vi "Triggers-Reset soft trigger.vi"(6 "Reset soft. trigger":bool, 8 "error in (no error)":errorcluster, 11 "FPGA Ref":T1) -> (0 "error out":errorcluster)   [LabVIEW 2013]
uses:
  RIG-SPECIFIC FILES/FPGA Refs/FPGA Ref.ctl
  <vilib>/rvi/interface/common/niFpgaWaitOnOcc.vi
  <vilib>/Utility/error.llb/Error Cluster From Error Code.vi
  <vilib>/rvi/errors/niLvFpgaAdjustHostInterfaceError.vi
  <vilib>/rvi/interface/nirviReadWriteControl/nirviReadWriteControl.xnode
  NiFpgaLv.dll
  <vilib>/rvi/interface/Simulation/niFpgaSimulationCallBeginRW.vi
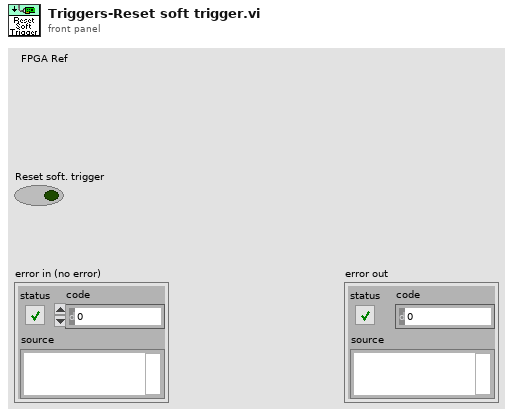
[diagram p1: front panel]
types:
  T1 = typedef "FPGA Ref.ctl" = refnum<k20>
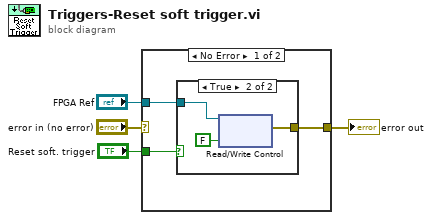
[diagram p0: block diagram]
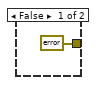
[diagram p2: hidden frame]
diagram:
  n1 = case shown="No Error" "error in (no error)" {
    selector: "error in (no error)" -> [_ w12]
    tunnel: [w5 w12] -> w4
    tunnel: "FPGA Ref" -> [w7 _]
    tunnel: "Reset soft. trigger" -> [w6 _]
    frame No Error {
      n2 = case shown="True" w6 {
        tunnel: w7 -> [_ w11]
        tunnel: [errorcluster {"status"=FALSE, "code"=0, "source"=""} ("error out") w9] -> w5
        frame False {
        }
        frame True {
          n3 = xnode "Read/Write Control"("FPGA VI Reference In"=w11, "start"=FALSE) -> ("error out"=w9:errorcluster)  [unwired: 1 in, 1 out]
        }
      }
    }
    frame Error {
    }
  }
  "error out" <- w4
